vi "Initialize.vi"(8 "error in (no error)":errorcluster, 11 "Sensor & Control in":refnum<class "Sensor & Control.lvclass">) -> (0 "error out":errorcluster, 3 "Sensor & Control out":refnum<class "Sensor & Control.lvclass">)   [LabVIEW 2013, in "Sensor & Control.lvlib" / "Sensor & Control.lvclass"]
uses:
  Sensor & Control.lvclass
  <vilib>/Instr/_visa.llb/VISA Flush IO Buffer Mask.ctl
  Sensor & Control.lvclass/Sensor & Control.ctl
  Read Setpoint.vi
  Read Value.vi
  Read Sampling Interval.vi
  Write VISA.vi
  <vilib>/Instr/_visa.llb/VISA Configure Serial Port (Instr).vi
  PluginInterface/PluginInterface.lvlibp/PluginInterfaceClass/Read Name.vi
  PluginInterface/PluginInterface.lvlibp/PluginInterfaceClass/Read TDMS File Path.vi
  PluginInterface/PluginInterface.lvlibp/PluginInterfaceClass/Read DVR.vi
  PluginInterface/PluginInterface.lvlibp/PluginInterfaceClass/Write TDMS.vi
  PluginInterface/Actor Framework.lvlibp/Stop Msg/Stop Msg.lvclass
  PluginInterface/Actor Framework.lvlibp/Actor/Actor.lvclass
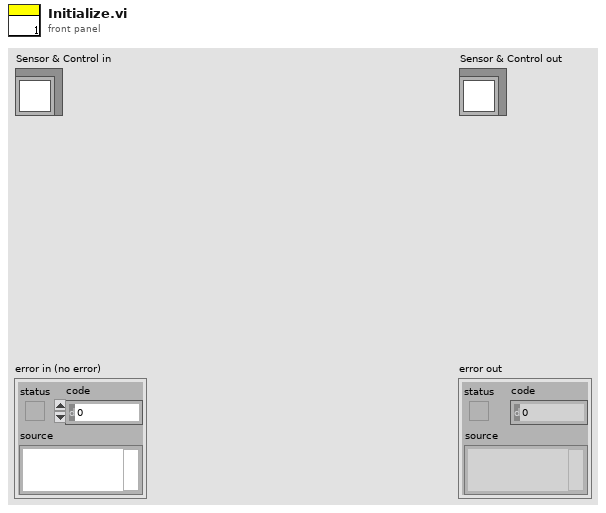
[diagram p1: front panel]
types:
  T1 = enum16{"open", "open or create", "create or replace", "create", "open (read-only)"}
  T2 = typedef "VISA Flush IO Buffer Mask.ctl" = u16
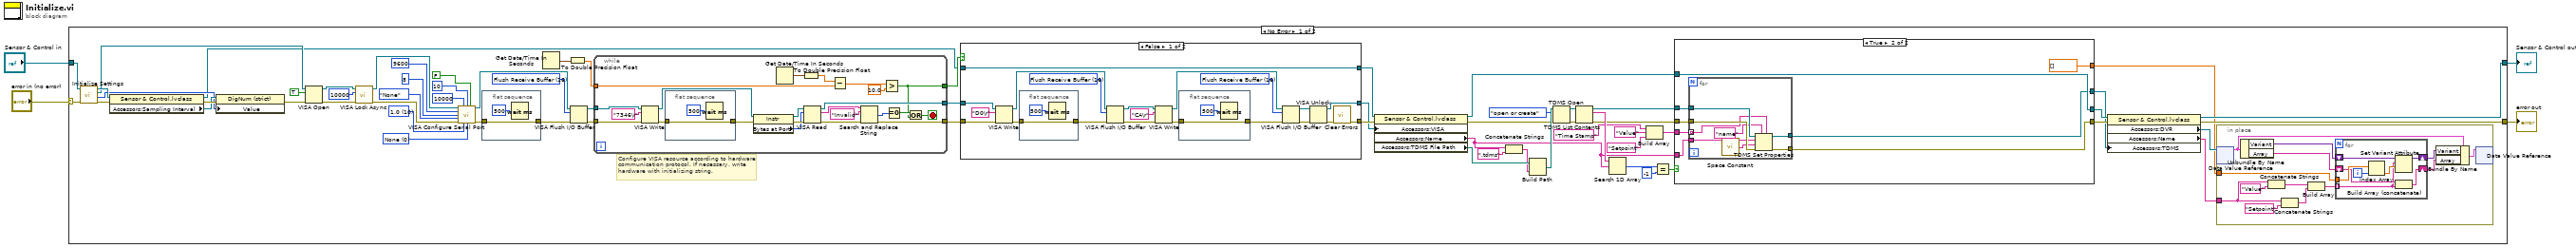
[diagram p0: block diagram]
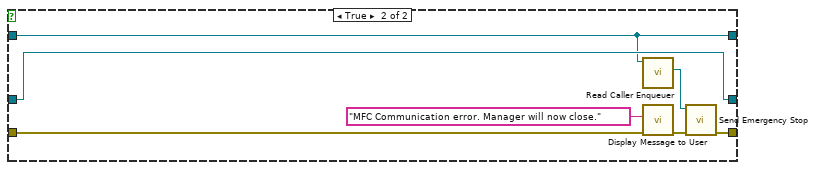
[diagram p2: hidden frame]
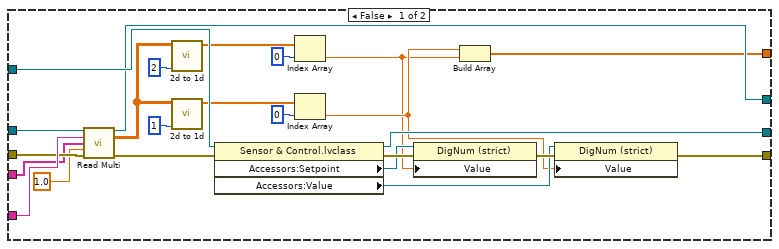
[diagram p3: hidden frame]
diagram:
  n1 = case shown="No Error" "error in (no error)" {
    selector: "error in (no error)" -> [w61 w191]
    tunnel: [w55 w191] -> w3
    tunnel: [w54 w190] -> w1
    tunnel: "Sensor & Control in" -> [w63 w190]
    frame No Error {
      w40 = T2 16 items=["Flush Receive Buffer"=16, "Write Transmit Buffer to Device"=32, "Flush Receive Buffer (No I/O)"=64, "Flush Transmit Buffer"=128] ("Mask")
      w43 = u16 0 items=["None", "XON/XOFF", "RTS/CTS", "XON/XOFF & RTS/CTS", "DTR/DSR", "XON/XOFF & DTR/DSR"] ("flow control (0:none)")
      w44 = u16 10 items=["1.0"=10, "1.5"=15, "2.0"=20] ("stop bits (10: 1 bit)")
      # "Configure VISA resource according to hardware\ncommunication protocol. If necessary, write\nhardware with initializing string."
      n2 = call "Initialize Settings.vi"("error in (no error)"=w61, "Sensor & Control in"=w63) -> ("error out"=w56:errorcluster, "Sampling Interval 2"=w58:i32, "VISA out"=w60:refnum<visa-resource-name>, "Sensor & Control out"=w62:refnum<class "Sensor & Control.lvclass">)  [unwired: 6 in]
      n3 = property class="Sensor & Control.lvclass"(reference=w62, error in=w56) -> (reference out=w6:refnum<class "Sensor & Control.lvclass">, error out=w64:errorcluster, "Accessors:Sampling Interval"=w59:refnum<vi>)
      n4 = property class="DigNum (strict)"(reference=w59, error in=w64, "Value"=w58) -> (error out=w57:errorcluster)  [unwired: 1 out]
      n5 = VISA Open(duplicate session (F)=TRUE, error in (no error)=w57, VISA resource name=w60) -> (VISA resource name=w66:refnum<visa-resource-name>, error out=w69:errorcluster)  [unwired: 2 in]
      n6 = call <vilib>:"VISA Lock Async.vi"("error in (no error)"=w69, "timeout (0)"=u32 10000, "VISA resource name"=w66) -> ("error out"=w68:errorcluster, "VISA resource name out"=w67:refnum<visa-resource-name>)  [unwired: 6 in, 1 out]
      n7 = call-poly "VISA Configure Serial Port"("VISA resource name"=w67, "timeout (10sec)"=u32 10000, "termination char\n(0xA = '\\n' = LF)"=u8 10 ("termination char\n(0xA = '\\n' = LF)"), "Enable Termination\nChar (T)"=FALSE ("Enable Termination\nChar (T)"), "baud rate (9600)"=u32 9600, "data bits (8)"=u16 8, "parity (0:none)"=enum16{"None", "Odd", "Even", "Mark", "Space"}."None", "error in (no error)"=w68, "stop bits (10: 1 bit)"=w44, "flow control (0:none)"=w43) -> ("VISA resource name out"=w39:refnum<visa-resource-name>, "error out"=w53:errorcluster)  [unwired: 4 in]
      n8 = flat-sequence {
        tunnel: w53 -> [w188]
        tunnel: [w188] -> w38
        frame #0 {
          n9 = Wait (ms)(milliseconds to wait=u32 500) -> ()  [unwired: 1 out]
        }
      }
      n10 = Get Date/Time In Seconds() -> (seconds since 1Jan1904=w42:timestamp)
      n11 = To Double Precision Float(number=w42) -> (double precision float=w41:dbl)
      n12 = VISA Flush I/O Buffer(VISA resource name=w39, mask (16)=w40, error in (no error)=w38) -> (VISA resource name out=w36:refnum<visa-resource-name>, error out=w37:errorcluster)
      n13 = while {
        tunnel: w37 -> [w170]
        tunnel: w36 -> [w182]
        tunnel: [w185] -> w49
        tunnel: [w184] -> w50
        tunnel: w41 -> [w168]
        tunnel: [w163] -> w7
        stop <- w164 stop-if-true
        n14 = VISA Write(VISA resource name=w182, write buffer="7346\r", error in (no error)=w170) -> (VISA resource name out=w180:refnum<visa-resource-name>, error out=w177:errorcluster)  [unwired: 1 out]
        n15 = flat-sequence {
          tunnel: [w186] -> w178
          tunnel: w177 -> [w186]
          frame #0 {
            n16 = Wait (ms)(milliseconds to wait=u32 500) -> ()  [unwired: 1 out]
          }
        }
        n17 = property class="Instr"(reference=w180, error in=w178) -> (reference out=w181:refnum<visa-resource-name>, error out=w179:errorcluster, "Bytes at Port"=w175:u32)
        n18 = Get Date/Time In Seconds() -> (seconds since 1Jan1904=w169:timestamp)
        n19 = To Double Precision Float(number=w169) -> (double precision float=w167:dbl)
        n20 = VISA Read(VISA resource name=w181, byte count=w175, error in (no error)=w179) -> (VISA resource name out=w184:refnum<visa-resource-name>, read buffer=w171:string, error out=w172:errorcluster)  [unwired: 1 out]
        n21 = Subtract(x=w167, y=w168) -> (x-y=w166:dbl)
        n22 = Search and Replace String(input string=w171, search string="Invalid", error in=w172) -> (number of replacements=w174:i32, error out=w185:errorcluster)  [unwired: 5 in, 2 out]
        n23 = Greater?(x=w166, y=10.0) -> (0:w163:bool)
        n24 = Equal To 0?(x=w174) -> (x = 0?=w183:bool)
        n25 = Or(x=w183, y=w163) -> (x .or. y?=w164:bool)
      }
      n26 = case shown="False" w7 {
        tunnel: w50 -> [w90 w101]
        tunnel: w49 -> [w89 w97]
        tunnel: [w88 w100] -> w25
        tunnel: [w86 w101] -> w16
        tunnel: w6 -> [w71 w99]
        tunnel: [w71 w99] -> w5
        frame False {
          w72 = T2 16 items=["Flush Receive Buffer"=16, "Write Transmit Buffer to Device"=32, "Flush Receive Buffer (No I/O)"=64, "Flush Transmit Buffer"=128] ("Mask")
          w77 = T2 16 items=["Flush Receive Buffer"=16, "Write Transmit Buffer to Device"=32, "Flush Receive Buffer (No I/O)"=64, "Flush Transmit Buffer"=128] ("Mask")
          n27 = VISA Write(VISA resource name=w90, write buffer="D0\r", error in (no error)=w89) -> (VISA resource name out=w78:refnum<visa-resource-name>, error out=w82:errorcluster)  [unwired: 1 out]
          n28 = flat-sequence {
            tunnel: [w93] -> w79
            tunnel: w82 -> [w93]
            frame #0 {
              n29 = Wait (ms)(milliseconds to wait=u32 500) -> ()  [unwired: 1 out]
            }
          }
          n30 = VISA Flush I/O Buffer(VISA resource name=w78, mask (16)=w77, error in (no error)=w79) -> (VISA resource name out=w75:refnum<visa-resource-name>, error out=w76:errorcluster)
          n31 = VISA Write(VISA resource name=w75, write buffer="CA\r", error in (no error)=w76) -> (VISA resource name out=w73:refnum<visa-resource-name>, error out=w80:errorcluster)  [unwired: 1 out]
          n32 = flat-sequence {
            tunnel: [w91] -> w74
            tunnel: w80 -> [w91]
            frame #0 {
              n33 = Wait (ms)(milliseconds to wait=u32 500) -> ()  [unwired: 1 out]
            }
          }
          n34 = VISA Flush I/O Buffer(VISA resource name=w73, mask (16)=w72, error in (no error)=w74) -> (VISA resource name out=w84:refnum<visa-resource-name>, error out=w85:errorcluster)
          n35 = VISA Unlock(8:w85, 11:w84) -> (0:w87:errorcluster, 3:w86:refnum<visa-resource-name>)
          n36 = call <vilib>:"Clear Errors.vi"("error in (no error)"=w87) -> ("error out"=w88:errorcluster)  [unwired: 6 in]
        }
        frame True {
          n37 = call "Read Caller Enqueuer.vi"("Actor"=w99) -> ("Caller Enqueuer"=w98:refnum<class "Message Enqueuer.lvclass">)  [unwired: 10 in]
          n38 = call "Display Message to User"("error in (no error)"=w97, "Message"="MFC Communication error. Manager will now close.") -> ("error out"=w96:errorcluster)  [unwired: 8 in, 1 out]
          n39 = call "Send Emergency Stop.vi"("error in (no error)"=w96, "Message Enqueuer"=w98) -> ("error out"=w100:errorcluster)  [unwired: 9 in]
        }
      }
      n40 = property class="Sensor & Control.lvclass"(reference=w5, error in=w25, "Accessors:VISA"=w16) -> (reference out=w9:refnum<class "Sensor & Control.lvclass">, error out=w8:errorcluster, "Accessors:Name"=w10:string, "Accessors:TDMS File Path"=w21:path)
      n41 = Concatenate Strings(w10, ".tdms" ("name or relative path")) -> (w12:string)
      n42 = Build Path(base path=w21, name or relative path=w12) -> (appended path=w24:path)
      n43 = TDMS Open(8:w8, 10:T1."open or create" ("operation (0:open)"), 11:w24) -> (0:w23:errorcluster, 3:w20:refnum<k34>)  [unwired: 4 in]
      n44 = TDMS List Contents(4:w23, 7:w20) -> (0:w30:errorcluster, 2:w33:string[], 3:w31:refnum<k34>)  [unwired: 1 in, 1 out]
      n45 = Search 1D Array(1D array=w33, element=w10) -> (index of element=w34:i32)  [unwired: 1 in]
      n46 = Build Array("Time Stamp" ("Channel"), "Value" ("string"), "Setpoint" ("string")) -> (w29:string[])
      n47 = Equal?(x=w34, y=-1) -> (x = y?=w32:bool)
      n48 = case shown="True" w32 {
        tunnel: w31 -> [w139 w154]
        tunnel: [w129 w150] -> w18
        tunnel: w30 -> [w142 w152]
        tunnel: w10 -> [w143 w153]
        tunnel: w9 -> [w146 w149]
        tunnel: w29 -> [w127 w151]
        tunnel: [w138 w149] -> w17
        tunnel: [w126 w148] -> w15
        tunnel: [w123 dbl[] []] -> w14
        frame False {
          n49 = call "Read Multi.vi"("tdms file in"=w139, "group"=w143, "Channel"=w127, "Numeric"=1.0, "error in (no error)"=w142) -> ("tdms file out"=w126:refnum<k34>, "Array"=w136:dbl[][], "error out"=w141:errorcluster)  [unwired: 7 in, 1 out]
          n50 = call "2d to 1d.vi"("index"=2, "array"=w136) -> ("output array"=w144:dbl[])  [unwired: 9 in]
          n51 = call "2d to 1d.vi"("index"=1, "array"=w136) -> ("output array"=w135:dbl[])  [unwired: 9 in]
          n52 = property class="Sensor & Control.lvclass"(reference=w146, error in=w141) -> (reference out=w138:refnum<class "Sensor & Control.lvclass">, error out=w134:errorcluster, "Accessors:Setpoint"=w132:refnum<vi>, "Accessors:Value"=w128:refnum<vi>)
          n53 = Index Array(array=w144, index=0) -> (element=w124:dbl)
          n54 = Index Array(array=w135, index=0) -> (element=w125:dbl)
          n55 = property class="DigNum (strict)"(reference=w132, error in=w134, "Value"=w124) -> (error out=w133:errorcluster)  [unwired: 1 out]
          n56 = Build Array(w125, w124) -> (w123:dbl[])
          n57 = property class="DigNum (strict)"(reference=w128, error in=w133, "Value"=w125) -> (error out=w129:errorcluster)  [unwired: 1 out]
        }
        frame True {
          n58 = for {
            tunnel: w152 -> [w162]
            tunnel: [w161] -> w150
            tunnel: w154 -> [w160]
            tunnel: w153 -> [w159]
            tunnel: w151 -> [w158] mode=indexing
            tunnel: [w155] -> w148
            n59 = call <vilib>:"Space Constant.vi"() -> ("String"=w156:string)
            n60 = TDMS Set Properties(5:w158, 7:"name" ("property names"), 8:w162, 9:w156, 10:w159, 11:w160) -> (0:w161:errorcluster, 3:w155:refnum<k34>)  [unwired: 2 out]
          }
        }
      }
      n61 = property class="Sensor & Control.lvclass"(reference=w17, error in=w18, "Accessors:TDMS"=w15) -> (reference out=w54:refnum<class "Sensor & Control.lvclass">, error out=w55:errorcluster, "Accessors:DVR"=w19:refnum<data-value>, "Accessors:Name"=w11:string)
      n62 = in-place {
        in-place-border: w14 -> [w109]
        in-place-border: w11 -> [w106]
        n63 = in-place-dvr #1(w19) -> (w111:cluster{"Array":string[], "Variant":variant})  [unwired: 1 out]
        n64 = Unbundle By Name(w111) -> ("Variant"=w113:variant, "Array"=w103:string[])
        n65 = Concatenate Strings(w106, "Value" ("string")) -> (w105:string)
        n66 = Concatenate Strings(w106, "Setpoint" ("string")) -> (w104:string)
        n67 = Build Array(w105, w104) -> (w110:string[])
        n68 = for {
          tunnel: w110 -> [w116] mode=indexing
          tunnel: w109 -> [w119]
          shift-right: [w121] -> w112
          shift-left: w113 -> [w122]
          shift-right: [w115] -> w102
          shift-left: w103 -> [w117]
          i -> [w120]
          n69 = Index Array(array=w119, index=w120) -> (element=w118:dbl)
          n70 = Set Variant Attribute(Variant=w122, name=w116, value=w118) -> (Variant out=w121:variant)  [unwired: 1 in, 2 out]
          n71 = Build Array (concatenate)(w117, w116) -> (w115:string[])
        }
        n72 = Bundle By Name(cluster=w111, "Variant"=w112, "Array"=w102) -> (w114:cluster{"Array":string[], "Variant":variant})
        n73 = in-place-dvr #1(w114) -> ()  [unwired: 2 out]
      }
    }
    frame Error {
    }
  }
  "error out" <- w3
  "Sensor & Control out" <- w1
